vi "LJstreamUD read config.vi"(0 "Working Directory":path, 5 "filename":string="ljstreamud.cfg", 7 "ChP Default":string="0#!#1#!#2#!#3#!#4#!#5#!#6#!#7#!#8#!#9#!#10#!#11#!#12#!#13#!#14#!#15#!#") -> (1 "Data File Prefix":string="data", 2 "Scan Rate (Hz)":dbl=500.0 format="%.3f", 3 "Graph History":i32=1000 min=0, 4 "# Channels":i32=4, 6 "Disable Scaling":bool, 8 "Max File Size (Bytes)":i32=1048576, 9 "Write To File":bool, 10 "Channel Setup":T1={"+Ch"=["0", "1", "2", "3", "4", "5", "6", "7"], "-Ch"=["199", "199", "199", "199", "199", "199", "199", "199"], "Ranges"=[0, 0, 0, 0, 0, 0, 0, 0], "Scaling Equation"=["y=v0", "y=v1", "y=v2", "y=v3", "y=v4", "y=v5", "y=v6", "y=v7"], "Graph?"=[]} {"Ranges" items=["LJ_rgBIP10V", "LJ_rgBIP5V", "LJ_rgUNI5V", "LJ_rgUNI2P5V", "LJ_rgUNI1P25V", "LJ_rgBIP1V", "LJ_rgUNIP625V", "LJ_rgBIPP1V", "LJ_rgBIPP01V"]}, 11 "Good Config":bool, 12 "Interval (ms)":u32=500, 13 "Resolution":u8, 14 "SettlingFactor":u8, 15 "error out":errorcluster)   [LabVIEW 2020]
uses:
  <vilib>/Utility/config.llb/Read Key (String).vi
  <vilib>/Utility/config.llb/Read Key (U32).vi
  <vilib>/Utility/config.llb/Read Key (Double).vi
  <vilib>/Utility/config.llb/Read Key (I32).vi
  <vilib>/Utility/config.llb/Read Key (Boolean).vi
  <vilib>/Utility/config.llb/NI_LVConfig.lvlib
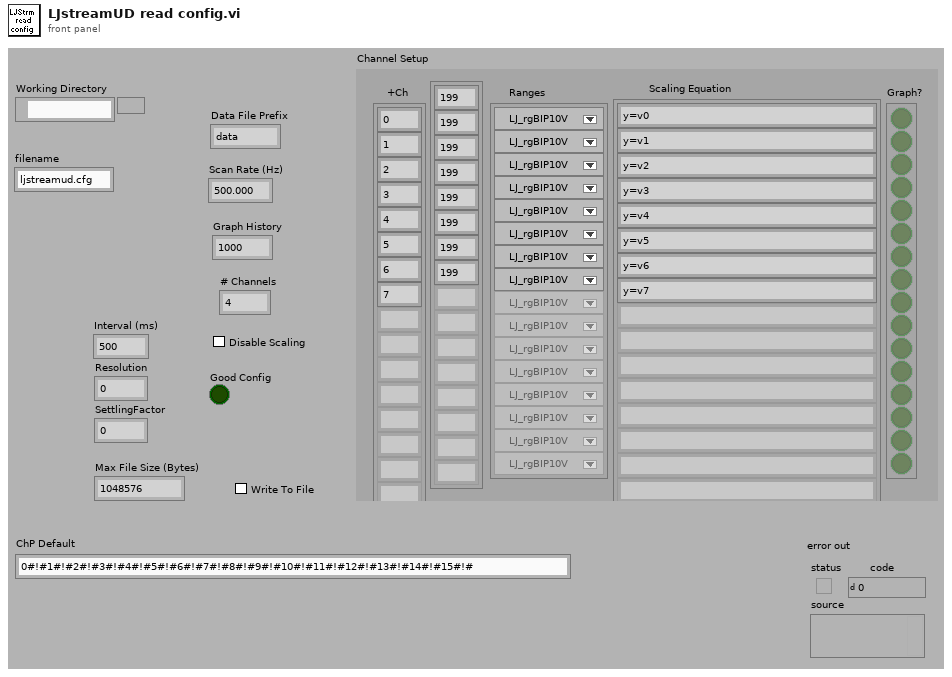
[diagram p1: front panel]
types:
  T1 = cluster{"+Ch":string[], "-Ch":string[], "Ranges":u16[], "Scaling Equation":string[], "Graph?":bool[]}
  T2 = typedef "NI_LVConfig.lvlib/Config Data RefNum.ctl" = refnum<k1>
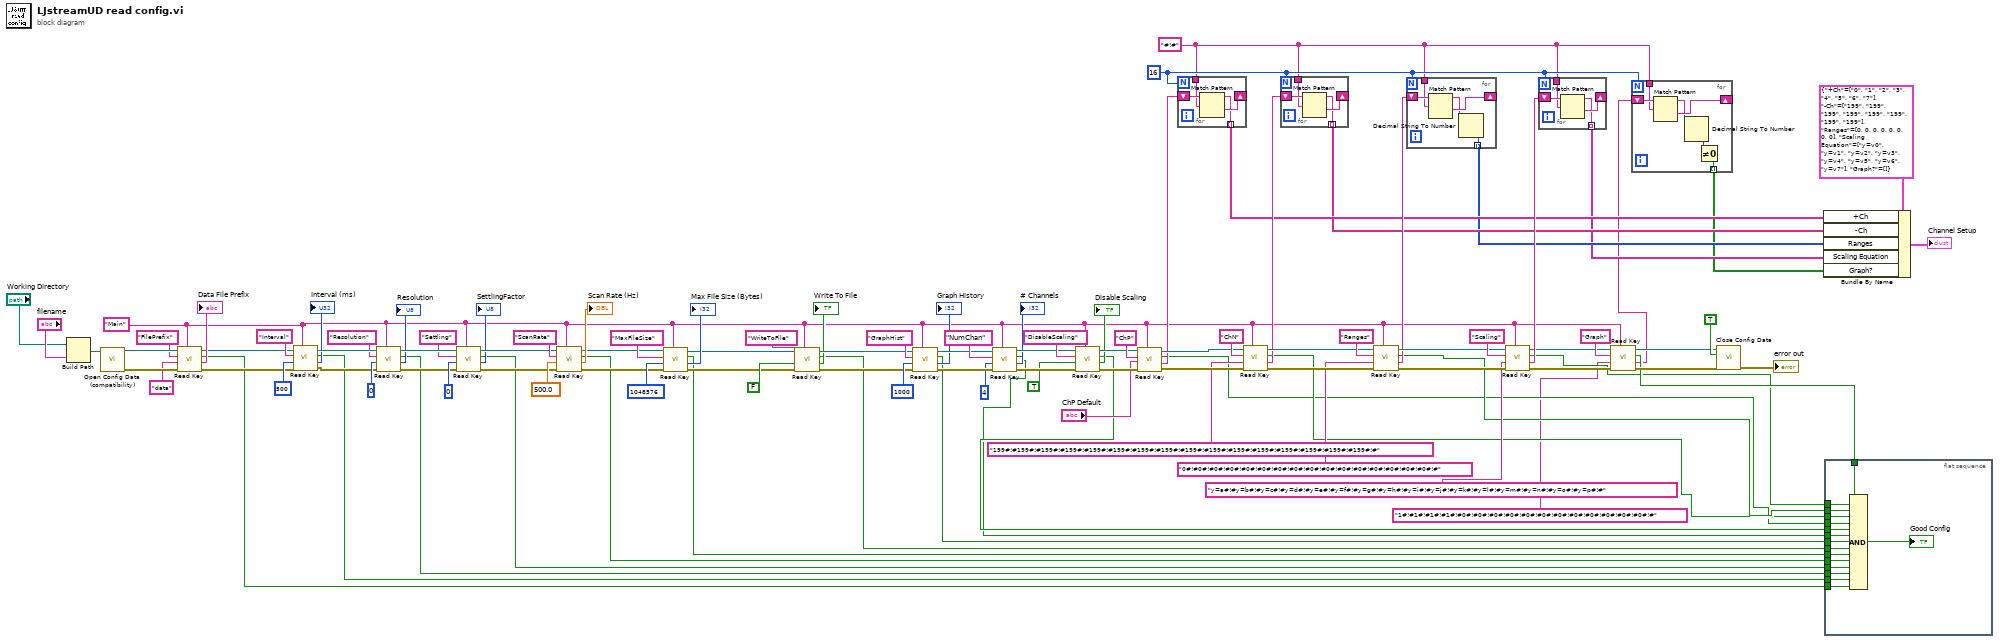
[diagram p0: block diagram]
diagram:
  w65 = 16
  w64 = "#!#" ("delimiter (Tab)")
  w18 = "Main" ("section")
  n1 = Build Path(base path="Working Directory", name or relative path="filename") -> (appended path=w106:path)
  n2 = call <vilib>:"Open Config Data (compatibility).vi"("configuration file path"=w106) -> ("error out"=w103:errorcluster, "refnum"=w104:T2)  [unwired: 8 in, 1 out]
  n3 = call-poly <vilib>:"Read Key.vi"("section"=w18, "error in (no error)"=w103, "default value"="data" ("Data File Prefix"), "key"="FilePrefix", "refnum"=w104) -> ("error out"=w39:errorcluster, "value"=→"Data File Prefix":string, "found?"=w3:bool, "refnum out"=w37:T2)  [unwired: 3 in]
  n4 = call-poly <vilib>:"Read Key.vi"("section"=w18, "error in (no error)"=w39, "default value"=u32 500 ("Scan Rate (Hz)"), "key"="Interval", "refnum"=w37) -> ("error out"=w44:errorcluster, "value"=→"Interval (ms)":u32, "found?"=w4:bool, "refnum out"=w43:T2)  [unwired: 3 in]
  n5 = call-poly <vilib>:"Read Key.vi"("section"=w18, "error in (no error)"=w44, "default value"=u8 0 ("Graph History"), "key"="Resolution", "refnum"=w43) -> ("error out"=w46:errorcluster, "value"=→"Resolution":u32, "found?"=w5:bool, "refnum out"=w45:T2)  [unwired: 3 in]
  n6 = call-poly <vilib>:"Read Key.vi"("section"=w18, "error in (no error)"=w46, "default value"=u8 0 ("# Channels"), "key"="Settling", "refnum"=w45) -> ("error out"=w38:errorcluster, "value"=→"SettlingFactor":u32, "found?"=w6:bool, "refnum out"=w36:T2)  [unwired: 3 in]
  n7 = call-poly <vilib>:"Read Key.vi"("section"=w18, "error in (no error)"=w38, "default value"=500.0 ("Scan Rate (Hz)"), "key"="ScanRate", "refnum"=w36) -> ("error out"=w29:errorcluster, "value"=→"Scan Rate (Hz)":dbl, "found?"=w7:bool, "refnum out"=w28:T2)  [unwired: 3 in]
  n8 = call-poly <vilib>:"Read Key.vi"("section"=w18, "error in (no error)"=w29, "default value"=1048576 ("Graph History"), "key"="MaxFileSize", "refnum"=w28) -> ("error out"=w22:errorcluster, "value"=→"Max File Size (Bytes)":i32, "found?"=w8:bool, "refnum out"=w23:T2)  [unwired: 3 in]
  n9 = call-poly <vilib>:"Read Key.vi"("section"=w18, "error in (no error)"=w22, "default value"=FALSE, "key"="WriteToFile", "refnum"=w23) -> ("error out"=w20:errorcluster, "value"=→"Write To File":bool, "found?"=w9:bool, "refnum out"=w21:T2)  [unwired: 3 in]
  n10 = call-poly <vilib>:"Read Key.vi"("section"=w18, "error in (no error)"=w20, "default value"=1000 ("Graph History"), "key"="GraphHist", "refnum"=w21) -> ("error out"=w98:errorcluster, "value"=→"Graph History":i32, "found?"=w10:bool, "refnum out"=w99:T2)  [unwired: 3 in]
  n11 = call-poly <vilib>:"Read Key.vi"("section"=w18, "error in (no error)"=w98, "default value"=4 ("# Channels"), "key"="NumChan", "refnum"=w99) -> ("error out"=w73:errorcluster, "value"=→"# Channels":i32, "found?"=w11:bool, "refnum out"=w74:T2)  [unwired: 3 in]
  n12 = call-poly <vilib>:"Read Key.vi"("section"=w18, "error in (no error)"=w73, "default value"=TRUE, "key"="DisableScaling", "refnum"=w74) -> ("error out"=w71:errorcluster, "value"=→"Disable Scaling":bool, "found?"=w12:bool, "refnum out"=w70:T2)  [unwired: 3 in]
  n13 = call-poly <vilib>:"Read Key.vi"("section"=w18, "error in (no error)"=w71, "default value"="ChP Default", "key"="ChP", "refnum"=w70) -> ("error out"=w93:errorcluster, "value"=w79:string, "found?"=w13:bool, "refnum out"=w94:T2)  [unwired: 3 in]
  n14 = for {
    N: w65 -> [_]
    shift-right: [w109] -> _
    shift-left: w79 -> [w111]
    tunnel: w64 -> [w110]
    tunnel: [w108] -> w55 mode=indexing
    n15 = Match Pattern(string=w111, regular expression=w110) -> (before substring=w108:string, after substring=w109:string)  [unwired: 1 in, 2 out]
  }
  n16 = call-poly <vilib>:"Read Key.vi"("section"=w18, "error in (no error)"=w93, "default value"="199#!#199#!#199#!#199#!#199#!#199#!#199#!#199#!#199#!#199#!#199#!#199#!#199#!#199#!#199#!#199#!#" ("Data File Prefix"), "key"="ChN", "refnum"=w94) -> ("error out"=w92:errorcluster, "value"=w78:string, "found?"=w14:bool, "refnum out"=w91:T2)  [unwired: 3 in]
  n17 = for {
    N: w65 -> [_]
    shift-right: [w113] -> _
    shift-left: w78 -> [w115]
    tunnel: w64 -> [w114]
    tunnel: [w112] -> w54 mode=indexing
    n18 = Match Pattern(string=w115, regular expression=w114) -> (before substring=w112:string, after substring=w113:string)  [unwired: 1 in, 2 out]
  }
  n19 = call-poly <vilib>:"Read Key.vi"("section"=w18, "error in (no error)"=w92, "default value"="0#!#0#!#0#!#0#!#0#!#0#!#0#!#0#!#0#!#0#!#0#!#0#!#0#!#0#!#0#!#0#!#" ("Data File Prefix"), "key"="Ranges", "refnum"=w91) -> ("error out"=w89:errorcluster, "value"=w77:string, "found?"=w15:bool, "refnum out"=w88:T2)  [unwired: 3 in]
  n20 = for {
    N: w65 -> [_]
    shift-right: [w118] -> _
    shift-left: w77 -> [w120]
    tunnel: w64 -> [w119]
    tunnel: [w116] -> w53 mode=indexing
    n21 = Match Pattern(string=w120, regular expression=w119) -> (before substring=w117:string, after substring=w118:string)  [unwired: 1 in, 2 out]
    n22 = Decimal String To Number(string=w117) -> (number=w116:i32)  [unwired: 2 in, 1 out]
  }
  n23 = call-poly <vilib>:"Read Key.vi"("section"=w18, "error in (no error)"=w89, "default value"="y=a#!#y=b#!#y=c#!#y=d#!#y=e#!#y=f#!#y=g#!#y=h#!#y=i#!#y=j#!#y=k#!#y=l#!#y=m#!#y=n#!#y=o#!#y=p#!#" ("Data File Prefix"), "key"="Scaling", "refnum"=w88) -> ("error out"=w68:errorcluster, "value"=w76:string, "found?"=w16:bool, "refnum out"=w63:T2)  [unwired: 3 in]
  n24 = for {
    N: w65 -> [_]
    shift-right: [w122] -> _
    shift-left: w76 -> [w124]
    tunnel: w64 -> [w123]
    tunnel: [w121] -> w52 mode=indexing
    n25 = Match Pattern(string=w124, regular expression=w123) -> (before substring=w121:string, after substring=w122:string)  [unwired: 1 in, 2 out]
  }
  n26 = call-poly <vilib>:"Read Key.vi"("section"=w18, "error in (no error)"=w68, "default value"="1#!#1#!#1#!#1#!#0#!#0#!#0#!#0#!#0#!#0#!#0#!#0#!#0#!#0#!#0#!#0#!#" ("Data File Prefix"), "key"="Graph", "refnum"=w63) -> ("error out"=w67:errorcluster, "value"=w2:string, "found?"=w17:bool, "refnum out"=w66:T2)  [unwired: 3 in]
  n27 = for {
    N: w65 -> [_]
    shift-right: [w128] -> _
    shift-left: w2 -> [w130]
    tunnel: w64 -> [w129]
    tunnel: [w125] -> w51 mode=indexing
    n28 = Match Pattern(string=w130, regular expression=w129) -> (before substring=w127:string, after substring=w128:string)  [unwired: 1 in, 2 out]
    n29 = Decimal String To Number(string=w127) -> (number=w126:i32)  [unwired: 2 in, 1 out]
    n30 = Not Equal To 0?(x=w126) -> (x != 0?=w125:bool)
  }
  n31 = call <vilib>:"Close Config Data.vi"("error in (no error)"=w67, "write file if changed (T)"=TRUE ("write configuration file? (F)"), "refnum"=w66) -> ("error out"=→"error out":errorcluster)  [unwired: 7 in, 1 out]
  n32 = Bundle By Name(cluster=T1 {"+Ch"=["0", "1", "2", "3", "4", "5", "6", "7"], "-Ch"=["199", "199", "199", "199", "199", "199", "199", "199"], "Ranges"=[0, 0, 0, 0, 0, 0, 0, 0], "Scaling Equation"=["y=v0", "y=v1", "y=v2", "y=v3", "y=v4", "y=v5", "y=v6", "y=v7"], "Graph?"=[]} ("Channel Setup"), "+Ch"=w55, "-Ch"=w54, "Ranges"=w53, "Scaling Equation"=w52, "Graph?"=w51) -> (→"Channel Setup":T1)
  n33 = flat-sequence {
    tunnel: w17 -> [w146]
    tunnel: w16 -> [w145]
    tunnel: w15 -> [w144]
    tunnel: w14 -> [w143]
    tunnel: w13 -> [w142]
    tunnel: w12 -> [w141]
    tunnel: w11 -> [w140]
    tunnel: w10 -> [w139]
    tunnel: w9 -> [w138]
    tunnel: w8 -> [w137]
    tunnel: w7 -> [w136]
    tunnel: w6 -> [w135]
    tunnel: w5 -> [w134]
    tunnel: w4 -> [w133]
    tunnel: w3 -> [w132]
    frame #0 {
      n34 = Compound Arithmetic op=AND(w146, w145, w144, w143, w142, w141, w140, w139, w138, w137, w136, w135, w134, w133, w132) -> (→"Good Config":bool)
    }
  }
